vi "fgt get sensor Range.vi"(8 "error in (no error)":errorcluster, 11 "sensorIndex":u32) -> (0 "error out":errorcluster, 2 "Smax out":sgl, 3 "Smin out":sgl)   [LabVIEW 2016, in "fgt_SDK.lvlib"]
doc: "Get sensor minimum and maximum range. Returned values takes into account set unit, default value is 'µl/min' in case of flow-units."
uses:
  fgt_SDK.lvlib
  dlls/fgt_SDK_32.dll
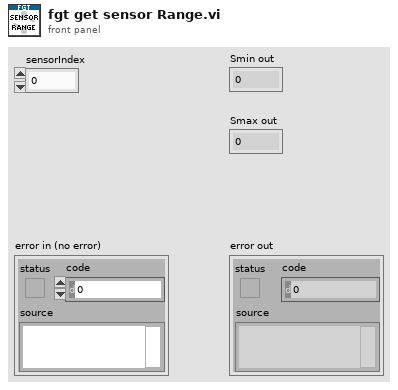
[diagram p1: front panel]
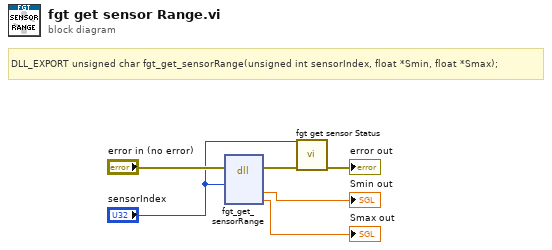
[diagram p0: block diagram]
diagram:
  # "DLL_EXPORT unsigned char fgt_get_sensorRange(unsigned int sensorIndex, float *Smin, float *Smax);"
  n1 = dll-call lib="PTH2Zabs D\nMes DocumentsDéveloppementFluigentSDKsfgt-sdk-labviewdllsfgt_SDK_*.*" fn="fgt_get_sensorRange"(error in="error in (no error)", "sensorIndex"="sensorIndex") -> (error out=w3:errorcluster, "Smin"=→"Smin out":sgl, "Smax"=→"Smax out":sgl)  [unwired: 6 in, 1 out]
  n2 = call "fgt get sensor Status.vi"("error in (no error)"=w3, "pressureIndex"="sensorIndex") -> ("error out"=→"error out":errorcluster)  [unwired: 9 in]
